vi "RT Main.vi"() -> ()   [LabVIEW 2018]
uses:
  Type Def Ctrls/RT ctrls/data summary.ctl
  <vilib>/Utility/error.llb/Error Cluster From Error Code.vi
  <vilib>/rvi/errors/niLvFpgaAdjustHostInterfaceError.vi
  <vilib>/rvi/interface/nirviReadWriteControl/nirviReadWriteControl.xnode
  Support/Message Queue/Message Queue.lvlib
  NiFpgaLv.dll
  <vilib>/rvi/interface/Simulation/niFpgaSimulationCallBeginRW.vi
panel:
  out "REQUEST_ID RESPONSE":u64
  out "REQUEST_ID INPUT":u64
  in  "connection parameters":T1={"baud rate (9600)"=115200, "data bits (8)"=8, "stop bits (10: 1 bit)"=10, "parity (0:none)"=enum."None", "flow control (0:none)"=0, "timeout (10sec)"=5000, "Enable Termination\nChar (T)"=TRUE, "termination char\n(0xA = '\\n' = LF)\n(0xD = '\\r' = CF) "=13} {"stop bits (10: 1 bit)" items=["1.0"=10, "1.5"=15, "2.0"=20]; "flow control (0:none)" items=["None", "XON/XOFF", "RTS/CTS", "XON/XOFF & RTS/CTS", "DTR/DSR", "XON/XOFF & DTR/DSR"]}
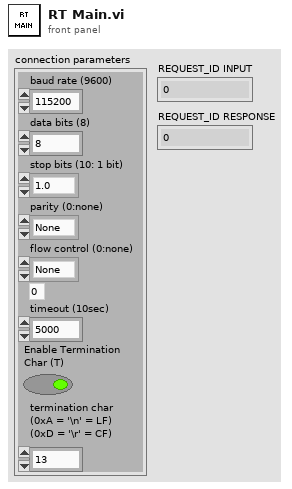
[diagram p1: front panel]
types:
  T1 = cluster{"baud rate (9600)":u32, "data bits (8)":u16, "stop bits (10: 1 bit)":u16, "parity (0:none)":enum16{"None", "Odd", "Even", "Mark", "Space"}, "flow control (0:none)":u16, "timeout (10sec)":u32, "Enable Termination\nChar (T)":bool, "termination char\n(0xA = '\\n' = LF)\n(0xD = '\\r' = CF) ":u8}
  T2 = typedef "data summary.ctl" = cluster{"TIMESTAMP":dbl, "INPUT_CHN_DATA":sgl[], "OUTPUT_CHN_DATA":sgl[], "CJC_TEMPERATURE":sgl, "RELAY_SETTING":u32, "REQUEST_ID":u64, "update_system_status?":bool, "update_error_log?":bool}
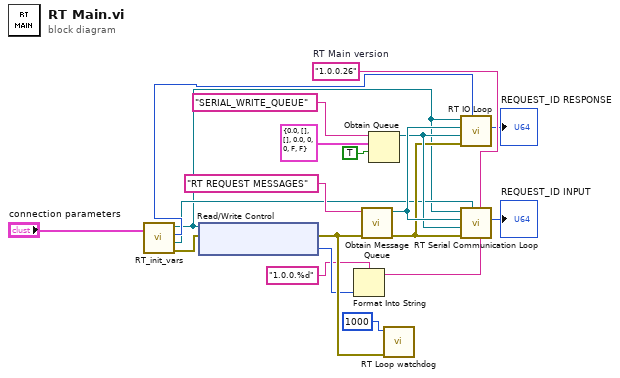
[diagram p0: block diagram]
diagram:
  w10 = "1.0.0.26"  # RT Main version
  n1 = call "RT_init_vars.vi"("connection parameters"="connection parameters") -> ("FPGA VI Reference Out"=w8:refnum<k20>, "FPGA I/O IRQ Number(s)"=w16:i32, "port name out"=w12:refnum<visa-resource-name>, "error out"=w7:errorcluster)  [unwired: 1 in]
  n2 = xnode "Read/Write Control"("FPGA VI Reference In"=w8, "error in"=w7) -> ("error out"=w6:errorcluster, "FPGA build Version"=w5:i16)  [unwired: 1 out]
  n3 = Format Into String(format string="1.0.0.%d", w5) -> (resulting string=w3:string)  [unwired: 2 in, 1 out]
  n4 = call "Obtain Message Queue.vi"("error in (no error)"=w6, "name (unnamed)"="RT REQUEST MESSAGES") -> ("error out"=w13:errorcluster, "Message Queue"=w15:refnum<queue>)  [unwired: 7 in, 1 out]
  n5 = Obtain Queue(name (unnamed)="SERIAL_WRITE_QUEUE", element data type=T2 {"TIMESTAMP"=0.0, "INPUT_CHN_DATA"=[], "OUTPUT_CHN_DATA"=[], "CJC_TEMPERATURE"=0.0, "RELAY_SETTING"=0, "REQUEST_ID"=0, "update_system_status?"=FALSE, "update_error_log?"=FALSE} ("data summary"), create if not found? (T)=TRUE) -> (queue out=w14:refnum<queue>)  [unwired: 2 in, 2 out]
  n6 = call "RT Loop watchdog.vi"("error in"=w6, "Watchdog pet rate (ms)"=u32 1000) -> ()  [unwired: 10 in]
  n7 = call "RT IO Loop.vi"("FPGA I/O IRQ Number(s)"=w16, "error in"=w13, "response queue"=w14, "message queue"=w15, "FPGA VI Reference in"=w8) -> ("REQUEST_ID"=→"REQUEST_ID RESPONSE":u64)  [unwired: 6 in]
  n8 = call "RT Serial Communication Loop.vi"("FPGA version"=w3, "RT Main version"=w10, "port name in"=w12, "error in"=w13, "response queue"=w14, "message queue"=w15, "FPGA VI Reference in"=w8) -> ("REQUEST_ID"=→"REQUEST_ID INPUT":u64)  [unwired: 4 in]
